vi "OpenCVLib_DetectFaces.vi"(8 "error in (no error)":errorcluster, 10 "Faces In":T1[](array[typedef]) {"Rotation" format="%.2f"; "Left" scale=0.0..1024.0; "Right" scale=0.0..1024.0}, 11 "Image Src":T2) -> (0 "error out":errorcluster, 2 "Faces":T1[](array[typedef]) {"Rotation" format="%.2f"; "Left" scale=0.0..1024.0; "Right" scale=0.0..1024.0}, 3 "Image Dst Out":T2)   [LabVIEW 2019]
doc: "<b> NIVisOpenCV FaceDetection</b> is a sample VI to use OpenCV Face Detection algorithm"
uses:
  <vilib>/vision/Image Controls.llb/IMAQ Image.ctl
  Binaries/Release/niopencvwrapper.dll
panel:
  out "Eyes":T1[](array[typedef]) {"Rotation" format="%.2f"; "Left" scale=0.0..1024.0; "Right" scale=0.0..1024.0}
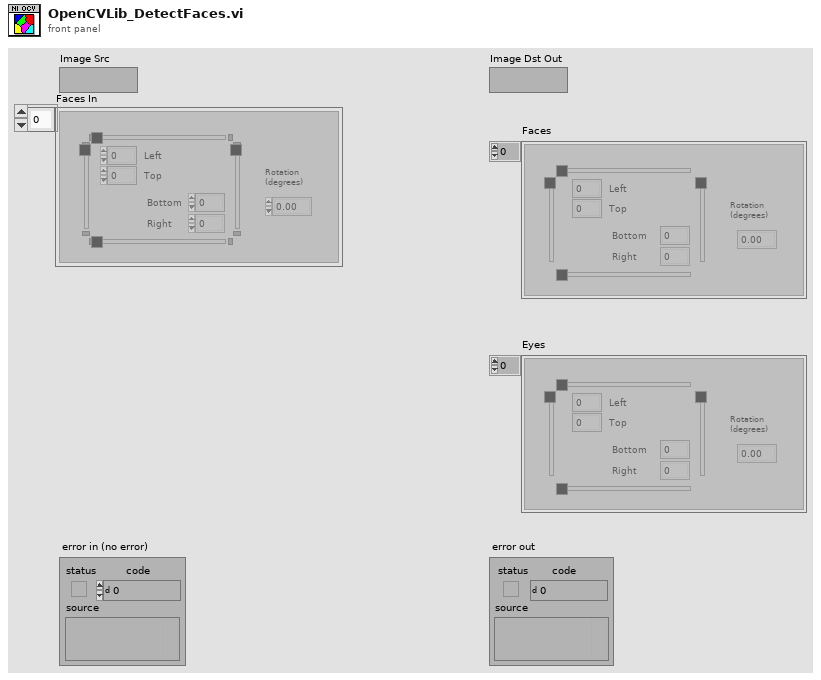
[diagram p1: front panel]
types:
  T1 = typedef "IMAQ Rectangle" = cluster{"Left":i32, "Top":i32, "Right":i32, "Bottom":i32, "Rotation":dbl}
  T2 = typedef "IMAQ Image.ctl" = refnum<image>
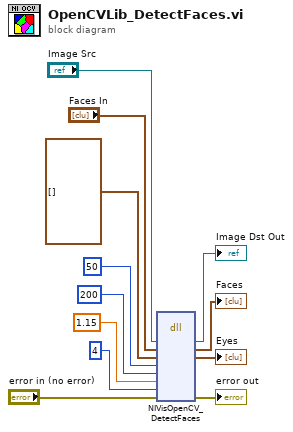
[diagram p0: block diagram]
diagram:
  n1 = dll-call lib="E:/Licenta/trip-validation-system/Binaries/Release/niopencvwrapper.dll" fn="NIVisOpenCV_DetectFaces"("Image Src"="Image Src", "faces"="Faces In", "eyes"=T1[] [] ("Eyes"), "minWidth"=50, "maxWidth"=200, "scaleFactor"=1.15, "minNeighbors"=4, "error"="error in (no error)") -> ("Image Src"=→"Image Dst Out":T2, "faces"=→"Faces":T1[], "eyes"=→"Eyes":T1[], "error"=→"error out":errorcluster)  [unwired: 8 in, 2 out]
